vi "filtrDecimace.vi"(6 "inicializace":bool, 11 "vstupniWaveform":waveform(dbl)) -> (0 "vzorkyPoDecimaci":i32, 1 "vzorkyPredDecimaci":i32, 3 "vystupniWaveform":waveform(dbl))   [LabVIEW 2018]
uses:
  <vilib>/Analysis/3filter.llb/Butterworth Filter (DBL).vi
  <vilib>/Analysis/NI_AALBase.lvlib
panel:
  out "pp":waveform(dbl)
  # "Vstupy:"
  # "Výstupy:"
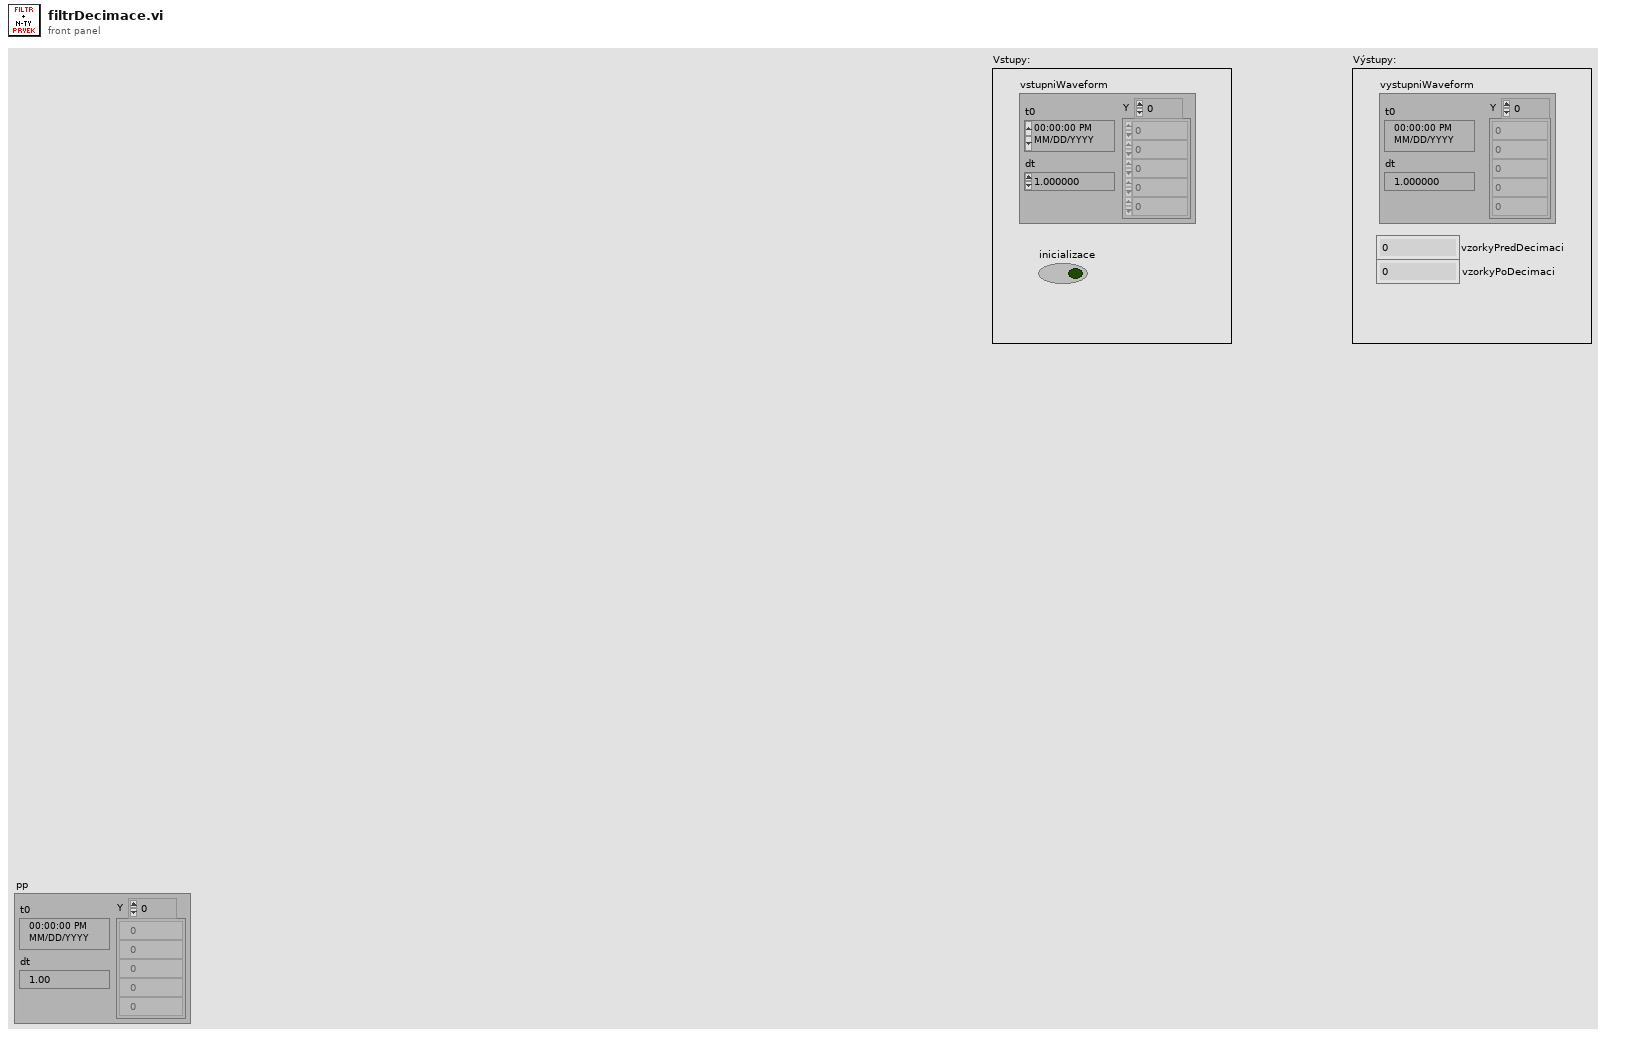
[diagram p1: front panel]
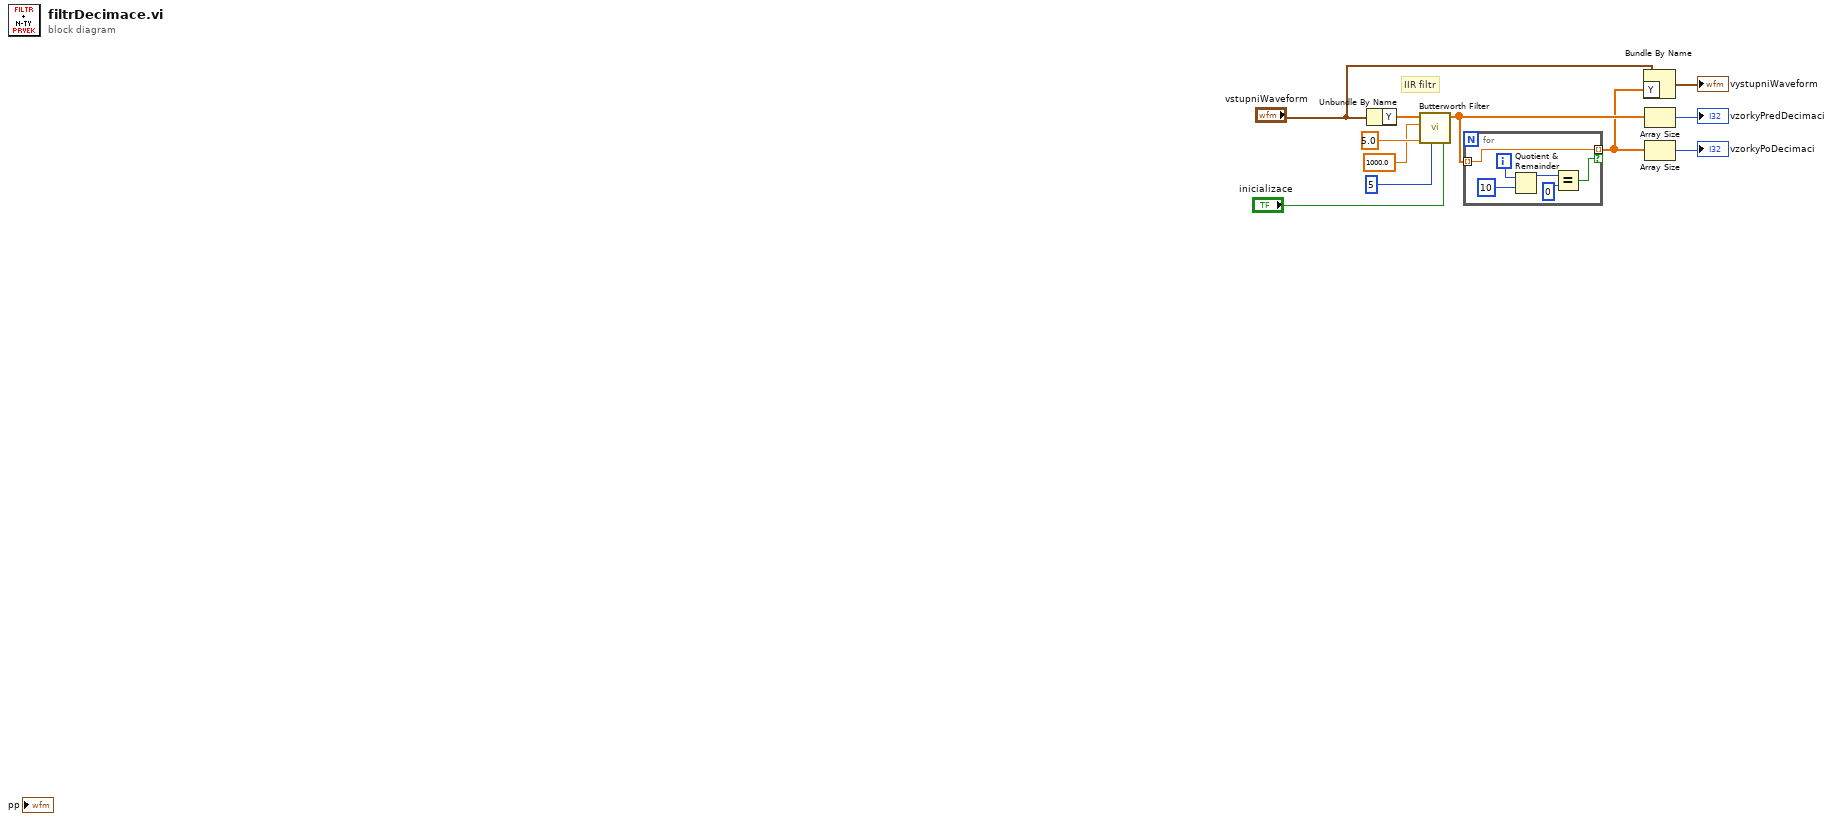
[diagram p0: block diagram]
diagram:
  # "IIR filtr"
  n1 = Unbundle By Name("vstupniWaveform") -> ("Y"=w9:dbl[])
  n2 = call-poly <vilib>:"Butterworth Filter.vi"("init/cont (init:F)"="inicializace", "order"=5, "low cutoff freq: fl"=5.0, "sampling freq: fs"=1000.0, "X"=w9) -> ("Filtered X"=w6:dbl[])  [unwired: 3 in, 1 out]
  n3 = for {
    tunnel: [w12] -> w3 mode=indexing if=w13
    tunnel: w6 -> [w12] mode=indexing
    i -> [w14]
    n4 = Quotient & Remainder(x=w14, y=10) -> (x-y*floor(x/y)=w16:i32)  [unwired: 1 out]
    n5 = Equal?(x=w16, y=0) -> (x = y?=w13:bool)
  }
  n6 = Bundle By Name(cluster="vstupniWaveform", "Y"=w3) -> (→"vystupniWaveform":waveform(dbl))
  n7 = Array Size(array=w6) -> (size(s)=→"vzorkyPredDecimaci":i32)
  n8 = Array Size(array=w3) -> (size(s)=→"vzorkyPoDecimaci":i32)
